vi "Plot B-Spline.vi"() -> ()   [LabVIEW 2019]
panel:
  in  "clamp?":bool
  out "num pts":i32
  out "time":u32
  in  "percision":dbl=0.001
  in  "weights":dbl[](array[numeric])
  in  "knots":dbl[](array[numeric])
  in  "degree":u16=2
  in  "points":dbl[][](array[numeric])
  out "points":cluster{"spline":dbl[], "spline":dbl[]}
  out "Spline":cluster{dbl[], dbl[]}(graph)
  # "knot vector will be ignored if true"
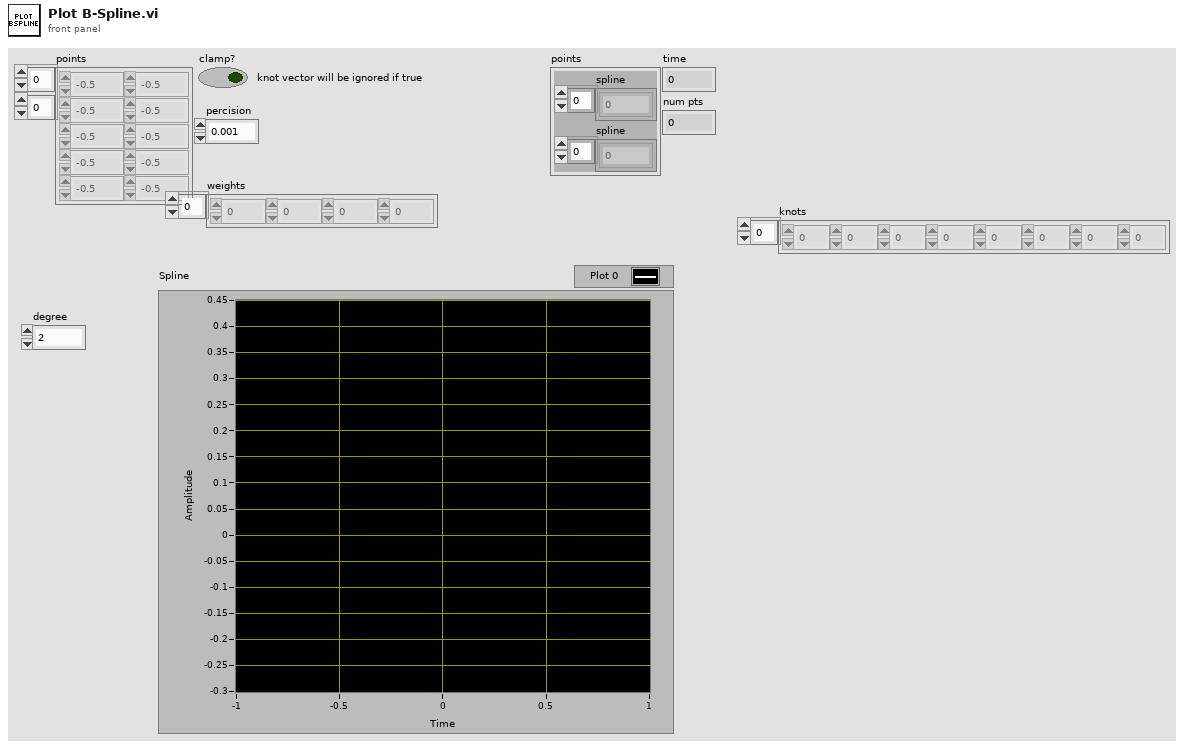
[diagram p1: front panel]
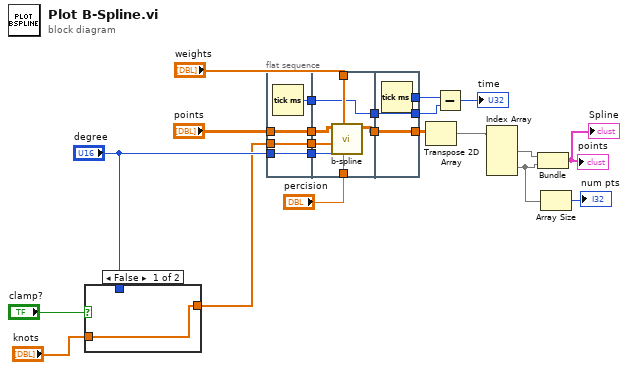
[diagram p0: block diagram]
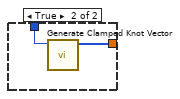
[diagram p2: hidden frame]
diagram:
  n1 = case shown="False" "clamp?" {
    tunnel: "degree" -> [_ w25]
    tunnel: [w23 w24] -> w1
    tunnel: "knots" -> [w23 _]
    frame False {
    }
    frame True {
      n2 = call "Generate Clamped Knot Vector.vi"("degree"=w25) -> ("knots"=w24:u32[])  [unwired: 9 in, 1 out]
    }
  }
  n3 = flat-sequence {
    tunnel: "degree" -> [w28]
    tunnel: "points" -> [w29]
    tunnel: [w29] -> w14
    tunnel: [w28] -> w13
    tunnel: [w27] -> w9
    tunnel: [w26] -> w2
    tunnel: w1 -> [w26]
    tunnel: "weights" -> [w34]
    tunnel: "percision" -> [w33]
    tunnel: [w32] -> w15
    tunnel: w14 -> [w36]
    tunnel: w13 -> [w35]
    tunnel: [w31] -> w10
    tunnel: w9 -> [w31]
    tunnel: w2 -> [w30]
    tunnel: [w39] -> w18
    tunnel: w15 -> [w39]
    tunnel: [w38] -> w12
    tunnel: [w37] -> w11
    tunnel: w10 -> [w37]
    frame #0 {
      n4 = Tick Count (ms)() -> (millisecond timer value=w27:u32)
    }
    frame #1 {
      n5 = call "b-spline.vi"("percision"=w33, "weights"=w34, "knots"=w30, "degree"=w35, "points"=w36) -> ("spline"=w32:dbl[][])  [unwired: 5 in, 1 out]
    }
    frame #2 {
      n6 = Tick Count (ms)() -> (millisecond timer value=w38:u32)
    }
  }
  n7 = Transpose 2D Array(2D array=w18) -> (transposed array=w17:dbl[][])
  n8 = Subtract(x=w12, y=w11) -> (x-y=→"time":u32)
  n9 = Index Array(array=w17) -> (element #1=w22:dbl[], element #2=w7:dbl[])  [unwired: 4 in]
  n10 = Bundle(w22, w7) -> (→"Spline" →"points":cluster{dbl[], dbl[]})  [unwired: 1 in]
  n11 = Array Size(array=w7) -> (size(s)=→"num pts":i32)
